vi "prop_axes_main.vi"() -> ()   [LabVIEW 2020, in "3DPC_SurfacePlot.xctl"]
uses:
  <vilib>/Native 3D Graph/xcontrol/3DPC_SurfacePlot.xctl
  <vilib>/Native 3D Graph/typedefs/prop_axes_all.ctl
  <vilib>/Native 3D Graph/typedefs/prop_axes_grid.ctl
  <vilib>/Native 3D Graph/typedefs/prop_axes_ticks.ctl
  <vilib>/Native 3D Graph/typedefs/range_cluster.ctl
  <vilib>/Native 3D Graph/typedefs/min_max.ctl
  <vilib>/Native 3D Graph/typedefs/prop_axes_captions.ctl
  <vilib>/Native 3D Graph/typedefs/prop_axes_labels.ctl
  <vilib>/Native 3D Graph/typedefs/prop_axes_autorange.ctl
  <vilib>/Utility/miscctls.llb/LVPointTypeDef.ctl
panel:
  in  "done":refnum<user-event>
  in  "quit":refnum<user-event>
  out "Axes Properties Out":T1
  in  "Axes Properties In":T1
  in  "Axes Listbox":i32(listbox) caption="Axes"
  in  "Tab Grid Prop":T9(tab)
  in  "Caption Opposite Visibility":bool
  in  "Caption Visibility":bool
  in  "Caption Font Size":i32 caption="Font Size"
  in  "Caption Color":u32(colorbox) caption="Color"
  in  "Caption Text":string
  in  "Label Opposite Visibility":bool
  in  "Label Color":u32(colorbox) caption="Color"
  in  "Label Font Size":i32 caption="Font Size"
  in  "Label Visibility":bool
  in  "Range Auto":bool
  in  "Range Minimum":dbl caption="Minimum"
  in  "Range Maximum":dbl caption="Maximum"
  in  "Grid Visibility":bool
  in  "Grid Color":u32(colorbox) caption="Color"
  in  "Major Tick Visibility":bool
  in  "Tick Color":u32(colorbox) caption="Color"
  in  "Major Tick Count":i32 caption="Count"
  in  "Minor Tick Visibility":bool
  in  "Minor Tick Count":i32 caption="Count"
  out "Boolean":bool caption="Major Ticks"
  out "Boolean 2":bool caption="Minor Ticks"
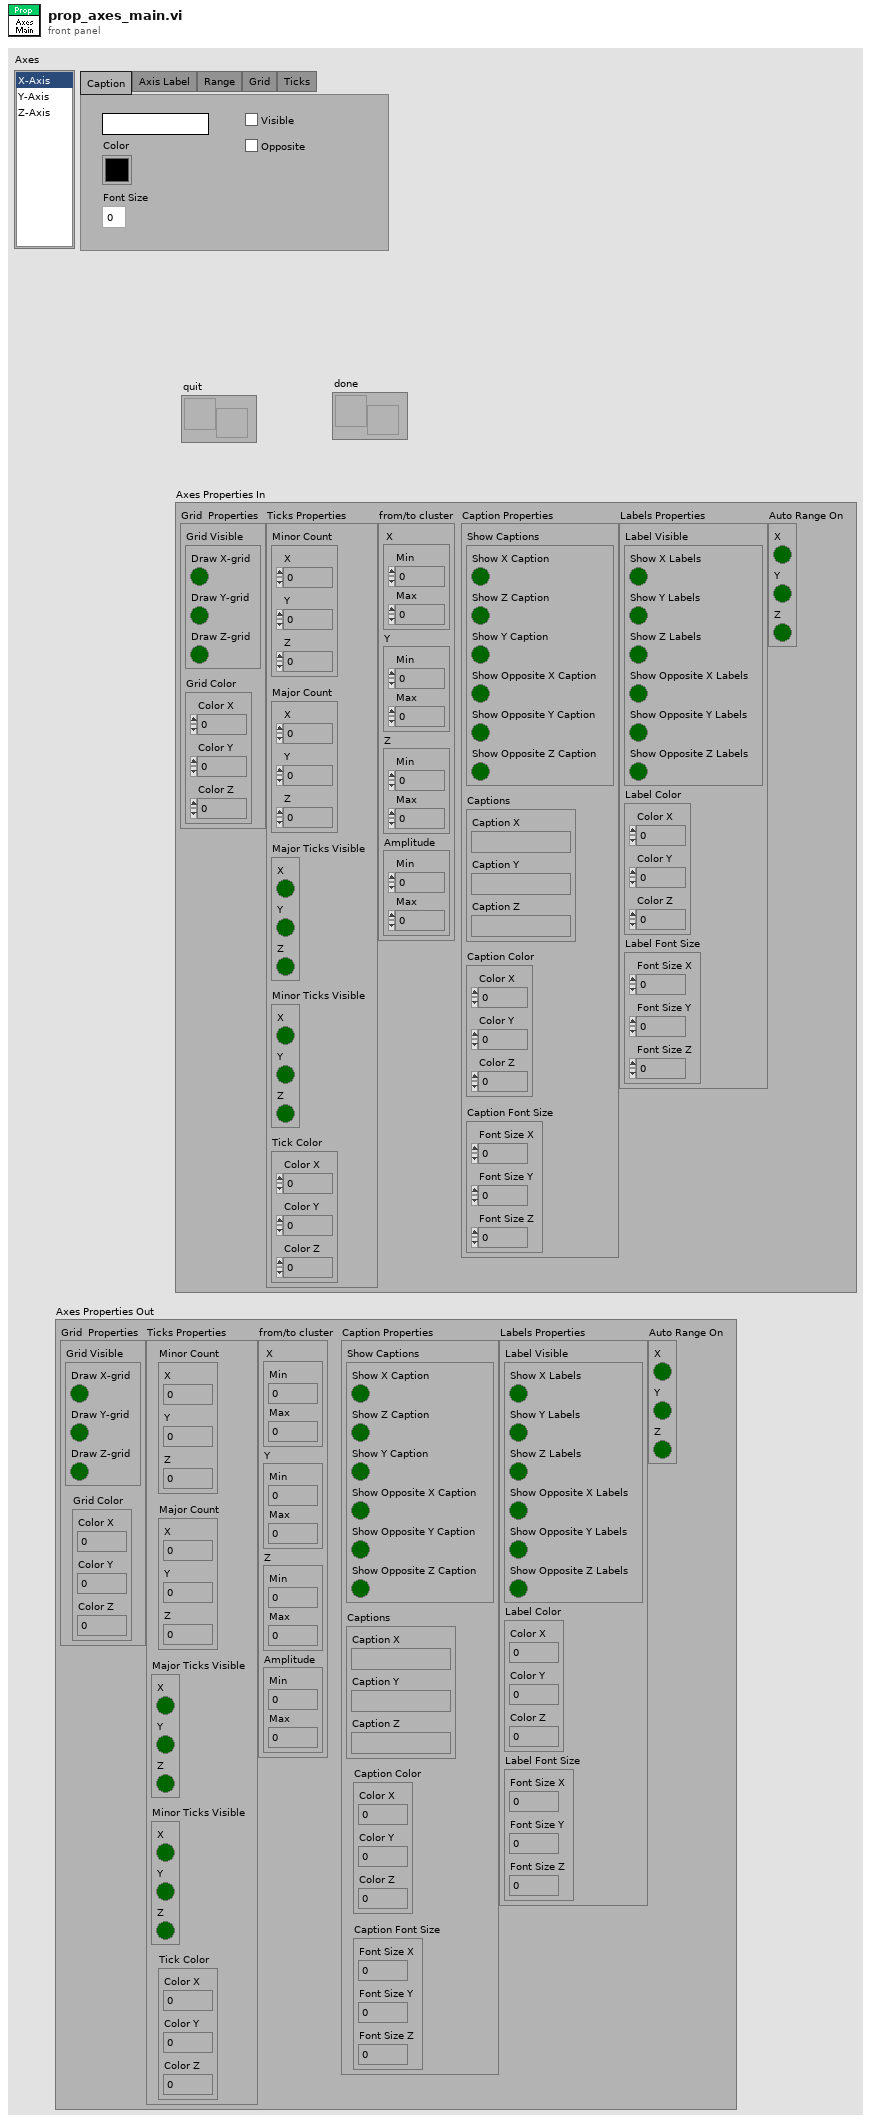
[diagram p1: front panel]
types:
  T1 = typedef "3DPC_SurfacePlot.xctl/prop_axes_all.ctl" = cluster{"Grid  Properties":T2, "Ticks Properties":T3, "from/to cluster":T4, "Caption Properties":T6, "Labels Properties":T7, "Auto Range On":T8}
  T2 = typedef "3DPC_SurfacePlot.xctl/prop_axes_grid.ctl" = cluster{"Grid Visible":cluster{"Draw X-grid":bool, "Draw Y-grid":bool, "Draw Z-grid":bool}, "Grid Color":cluster{"Color X":u32, "Color Y":u32, "Color Z":u32}}
  T3 = typedef "3DPC_SurfacePlot.xctl/prop_axes_ticks.ctl" = cluster{"Minor Count":cluster{"X":i32, "Y":i32, "Z":i32}, "Major Count":cluster{"X":i32, "Y":i32, "Z":i32}, "Major Ticks Visible":cluster{"X":bool, "Y":bool, "Z":bool}, "Minor Ticks Visible":cluster{"X":bool, "Y":bool, "Z":bool}, "Tick Color":cluster{"Color X":u32, "Color Y":u32, "Color Z":u32}}
  T4 = typedef "3DPC_SurfacePlot.xctl/range_cluster.ctl" = cluster{"X":T5, "Y":T5, "Z":T5, "Amplitude":T5}
  T5 = typedef "3DPC_SurfacePlot.xctl/min_max.ctl" = cluster{"Min":sgl, "Max":sgl}
  T6 = typedef "3DPC_SurfacePlot.xctl/prop_axes_captions.ctl" = cluster{"Show Captions":cluster{"Show X Caption":bool, "Show Z Caption":bool, "Show Y Caption":bool, "Show Opposite X Caption":bool, "Show Opposite Y Caption":bool, "Show Opposite Z Caption":bool}, "Captions":cluster{"Caption X":string, "Caption Y":string, "Caption Z":string}, "Caption Color":cluster{"Color X":u32, "Color Y":u32, "Color Z":u32}, "Caption Font Size":cluster{"Font Size X":i16, "Font Size Y":i16, "Font Size Z":i16}}
  T7 = typedef "3DPC_SurfacePlot.xctl/prop_axes_labels.ctl" = cluster{"Label Visible":cluster{"Show X Labels":bool, "Show Y Labels":bool, "Show Z Labels":bool, "Show Opposite X Labels":bool, "Show Opposite Y Labels":bool, "Show Opposite Z Labels":bool}, "Label Color":cluster{"Color X":u32, "Color Y":u32, "Color Z":u32}, "Label Font Size":cluster{"Font Size X":i16, "Font Size Y":i16, "Font Size Z":i16}}
  T8 = typedef "3DPC_SurfacePlot.xctl/prop_axes_autorange.ctl" = cluster{"X":bool, "Y":bool, "Z":bool}
  T9 = enum32{"Caption", "Axis Label", "Range", "Grid", "Ticks"}
  T10 = typedef "LVPointTypeDef.ctl" = cluster{"Horizontal":i16, "Vertical":i16}
  T11 = cluster{"Caption Properties":cluster{"Caption Visibility":bool, "Caption Opposite Visibility":bool, "Caption Color":u32, "Caption Font Size":i32, "Caption Text":string}, "Range Properties":cluster{"Range Auto":bool, "Range Maximum":dbl, "Range Minimum":dbl}, "Grid Properties":cluster{"Grid Visibility":bool, "Grid Color":u32}, "Minor Tick Properties":cluster{"Minor Tick Visibility":bool, "Minor Tick Count":i32}, "Major Tick Properties":cluster{"Major Tick Visibility":bool, "Major Tick Count":i32}, "Label Properties":cluster{"Label Visibility":bool, "Label Opposite Visibility":bool, "Label Color":u32, "Label Font Size":i32}, "Tick Color":u32}[]
  T12 = cluster{"Caption Properties":cluster{"Caption Visibility":bool, "Caption Opposite Visibility":bool, "Caption Color":u32, "Caption Font Size":i32, "Caption Text":string}, "Range Properties":cluster{"Range Auto":bool, "Range Maximum":dbl, "Range Minimum":dbl}, "Grid Properties":cluster{"Grid Visibility":bool, "Grid Color":u32}, "Minor Tick Properties":cluster{"Minor Tick Visibility":bool, "Minor Tick Count":i32}, "Major Tick Properties":cluster{"Major Tick Visibility":bool, "Major Tick Count":i32}, "Label Properties":cluster{"Label Visibility":bool, "Label Opposite Visibility":bool, "Label Color":u32, "Label Font Size":i32}, "Tick Color":u32}
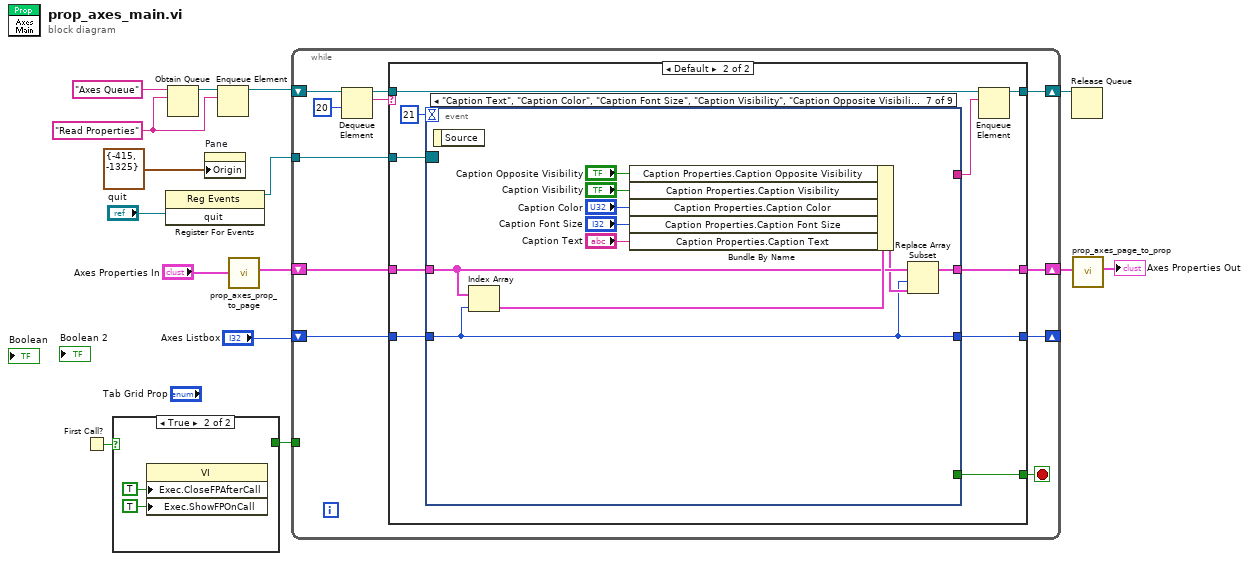
[diagram p0: block diagram]
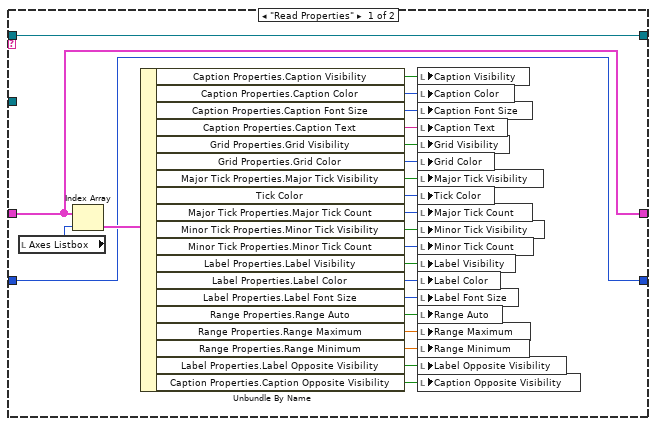
[diagram p2: hidden frame]
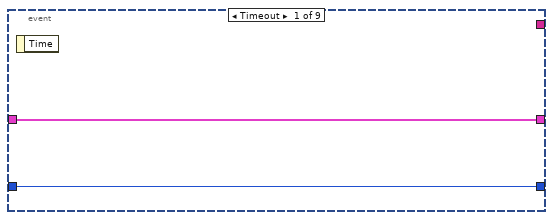
[diagram p3: hidden frame]
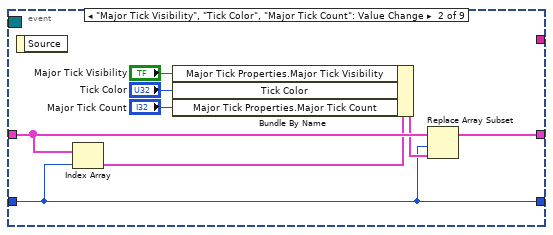
[diagram p4: hidden frame]
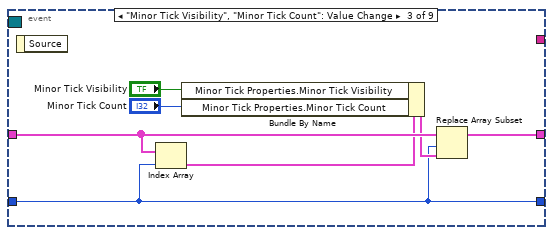
[diagram p5: hidden frame]
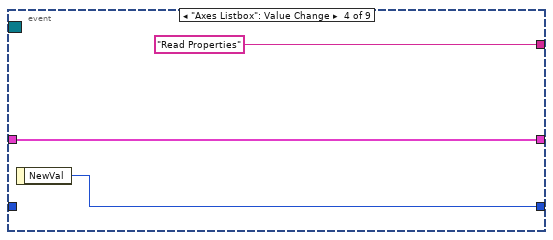
[diagram p6: hidden frame]
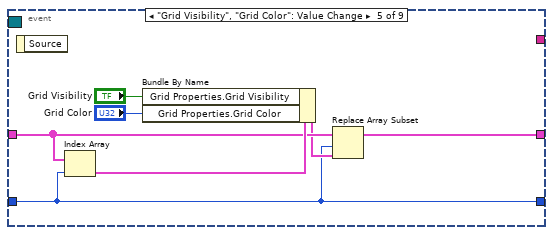
[diagram p7: hidden frame]
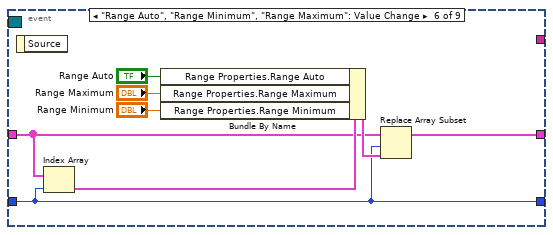
[diagram p8: hidden frame]
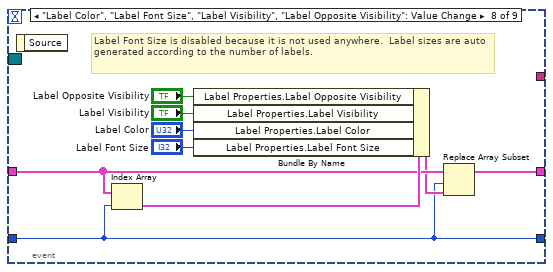
[diagram p9: hidden frame]
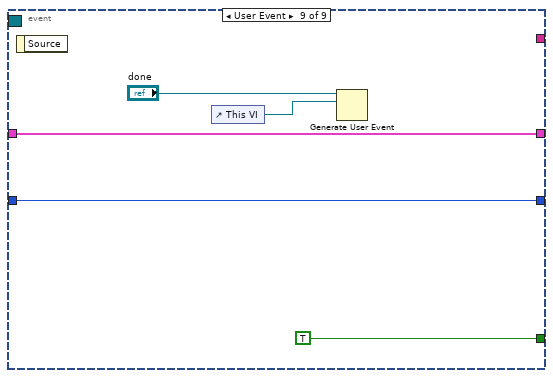
[diagram p10: hidden frame]
diagram:
  w13 = "Read Properties"
  n1 = First Call?() -> (First Call?: T/F=w1:bool)
  n2 = case shown="True" w1 {
    selector: w1 -> [w16 _]
    tunnel: [w16 _] -> w10
    frame False {
    }
    frame True {
      n3 = property class="VI"("Exec.CloseFPAfterCall"=TRUE ("Execution:Close After Call"), "Exec.ShowFPOnCall"=TRUE ("Execution:Show Front Panel On Call")) -> ()  [unwired: 2 in, 2 out]
    }
  }
  n4 = register-events("quit") -> (reference out=w4:refnum<event-registration>)  [unwired: 2 in, 1 out]
  n5 = Obtain Queue(name (unnamed)="Axes Queue", element data type=w13) -> (queue out=w14:refnum<queue>)  [unwired: 3 in, 2 out]
  n6 = property on="Pane" class="Pane"("Origin"=T10 {"Horizontal"=-415, "Vertical"=-1325} ("Point")) -> ()  [unwired: 2 in, 2 out]
  n7 = Enqueue Element(queue=w14, element=w13) -> (queue out=w12:refnum<queue>)  [unwired: 1 in, 3 out]
  n8 = call <vilib>:"prop_axes_prop_to_page.vi"("Axes Properties"="Axes Properties In") -> ("Axes Property Page"=w9:T11)  [unwired: 10 out]
  n9 = while {
    shift-right: [w28] -> w6
    shift-left: w9 -> [w29]
    shift-right: [w24] -> w11
    shift-left: w12 -> [w26]
    tunnel: w10 -> [_]
    tunnel: w4 -> [w22]
    shift-right: [w20] -> _
    shift-left: "Axes Listbox" -> [w19]
    stop <- w21 stop-if-true
    n10 = Dequeue Element(queue=w26, timeout in ms (-1)=20) -> (queue out=w25:refnum<queue>, element=w23:string)  [unwired: 1 in, 2 out]
    n11 = case shown="Default" w23 {
      tunnel: w29 -> [w31 w63]
      tunnel: [w31 w62] -> w28
      tunnel: w25 -> [w53 w60]
      tunnel: [w53 w61] -> w24
      tunnel: w22 -> [_ w57]
      tunnel: [_ w56] -> w21
      tunnel: [w30 w55] -> w20
      tunnel: w19 -> [w30 w54]
      frame "Read Properties" {
        n12 = local read "Axes Listbox"() -> (w32:i32)
        n13 = Index Array(array=w31, index=w32) -> (element=w52:T12)
        n14 = Unbundle By Name(w52) -> ("Caption Properties.Caption Visibility"=w51:bool, "Caption Properties.Caption Color"=w50:u32, "Caption Properties.Caption Font Size"=w49:i32, "Caption Properties.Caption Text"=w48:string, "Grid Properties.Grid Visibility"=w47:bool, "Grid Properties.Grid Color"=w46:u32, "Major Tick Properties.Major Tick Visibility"=w45:bool, "Tick Color"=w44:u32, "Major Tick Properties.Major Tick Count"=w43:i32, "Minor Tick Properties.Minor Tick Visibility"=w42:bool, "Minor Tick Properties.Minor Tick Count"=w41:i32, "Label Properties.Label Visibility"=w40:bool, "Label Properties.Label Color"=w39:u32, "Label Properties.Label Font Size"=w38:i32, "Range Properties.Range Auto"=w37:bool, "Range Properties.Range Maximum"=w36:dbl, "Range Properties.Range Minimum"=w35:dbl, "Label Properties.Label Opposite Visibility"=w34:bool, "Caption Properties.Caption Opposite Visibility"=w33:bool)
        n15 = local write "Caption Visibility"(w51) -> ()
        n16 = local write "Caption Color"(w50) -> ()
        n17 = local write "Caption Font Size"(w49) -> ()
        n18 = local write "Caption Text"(w48) -> ()
        n19 = local write "Grid Visibility"(w47) -> ()
        n20 = local write "Grid Color"(w46) -> ()
        n21 = local write "Major Tick Visibility"(w45) -> ()
        n22 = local write "Tick Color"(w44) -> ()
        n23 = local write "Major Tick Count"(w43) -> ()
        n24 = local write "Minor Tick Visibility"(w42) -> ()
        n25 = local write "Minor Tick Count"(w41) -> ()
        n26 = local write "Label Visibility"(w40) -> ()
        n27 = local write "Label Color"(w39) -> ()
        n28 = local write "Label Font Size"(w38) -> ()
        n29 = local write "Range Auto"(w37) -> ()
        n30 = local write "Range Maximum"(w36) -> ()
        n31 = local write "Range Minimum"(w35) -> ()
        n32 = local write "Label Opposite Visibility"(w34) -> ()
        n33 = local write "Caption Opposite Visibility"(w33) -> ()
      }
      frame Default {
        n34 = event shown="[6] \"Caption Text\", \"Caption Color\", \"Caption Font Size\", \"Caption Visibility\", \"Caption Opposite Visibility\": Value Change" {
          selector: w57 -> [_ _ _ _ _ _ _ _ _]
          dyn-events: _ -> [_ _ _ _ _ _ _ _ _]
          timeout: 21 -> [_ _ _ _ _ _ _ _ _]
          tunnel: w63 -> [w65 w72 w80 w82 w89 w91 w103 w113 w119]
          tunnel: [w65 w73 w75 w82 w88 w97 w101 w111 w119] -> w62
          tunnel: [_ _ _ "Read Properties" _ _ _ _ _] -> w59
          tunnel: [_ _ _ _ _ _ _ _ TRUE] -> w56
          tunnel: [w64 w67 w74 w81 w84 w92 w99 w109 w118] -> w55
          tunnel: w54 -> [w64 w67 w74 _ w84 w92 w99 w109 w118]
          event Timeout {
            n35 = event-data() -> ()  [unwired: 2 out]
          }
          event "Major Tick Visibility", "Tick Color", "Major Tick Count": Value Change {
            n36 = event-data() -> ()  [unwired: 2 out]
            n37 = Index Array(array=w72, index=w67) -> (element=w71:T12)
            n38 = Bundle By Name(cluster=w71, "Major Tick Properties.Major Tick Visibility"="Major Tick Visibility", "Tick Color"="Tick Color", "Major Tick Properties.Major Tick Count"="Major Tick Count") -> (w68:T12)
            n39 = Replace Array Subset(array=w72, new element=w68, index=w67) -> (w73:T11)
          }
          event "Minor Tick Visibility", "Minor Tick Count": Value Change {
            n40 = event-data() -> ()  [unwired: 2 out]
            n41 = Index Array(array=w80, index=w74) -> (element=w79:T12)
            n42 = Bundle By Name(cluster=w79, "Minor Tick Properties.Minor Tick Visibility"="Minor Tick Visibility", "Minor Tick Properties.Minor Tick Count"="Minor Tick Count") -> (w76:T12)
            n43 = Replace Array Subset(array=w80, new element=w76, index=w74) -> (w75:T11)
          }
          event "Axes Listbox": Value Change {
            n44 = event-data() -> ("NewVal"=w81:i32)  [unwired: 1 out]
          }
          event "Grid Visibility", "Grid Color": Value Change {
            n45 = event-data() -> ()  [unwired: 2 out]
            n46 = Index Array(array=w89, index=w84) -> (element=w90:T12)
            n47 = Bundle By Name(cluster=w90, "Grid Properties.Grid Visibility"="Grid Visibility", "Grid Properties.Grid Color"="Grid Color") -> (w87:T12)
            n48 = Replace Array Subset(array=w89, new element=w87, index=w84) -> (w88:T11)
          }
          event "Range Auto", "Range Minimum", "Range Maximum": Value Change {
            n49 = event-data() -> ()  [unwired: 2 out]
            n50 = Index Array(array=w91, index=w92) -> (element=w98:T12)
            n51 = Bundle By Name(cluster=w98, "Range Properties.Range Auto"="Range Auto", "Range Properties.Range Maximum"="Range Maximum", "Range Properties.Range Minimum"="Range Minimum") -> (w93:T12)
            n52 = Replace Array Subset(array=w91, new element=w93, index=w92) -> (w97:T11)
          }
          event "Caption Text", "Caption Color", "Caption Font Size", "Caption Visibility", "Caption Opposite Visibility": Value Change {
            n53 = event-data() -> ()  [unwired: 2 out]
            n54 = Index Array(array=w103, index=w99) -> (element=w104:T12)
            n55 = Bundle By Name(cluster=w104, "Caption Properties.Caption Opposite Visibility"="Caption Opposite Visibility", "Caption Properties.Caption Visibility"="Caption Visibility", "Caption Properties.Caption Color"="Caption Color", "Caption Properties.Caption Font Size"="Caption Font Size", "Caption Properties.Caption Text"="Caption Text") -> (w102:T12)
            n56 = Replace Array Subset(array=w103, new element=w102, index=w99) -> (w101:T11)
          }
          event "Label Color", "Label Font Size", "Label Visibility", "Label Opposite Visibility": Value Change {
            # "Label Font Size is disabled because it is not used anywhere.  Label sizes are auto generated according to the number of labels."
            n57 = event-data() -> ()  [unwired: 2 out]
            n58 = Index Array(array=w113, index=w109) -> (element=w117:T12)
            n59 = Bundle By Name(cluster=w117, "Label Properties.Label Opposite Visibility"="Label Opposite Visibility", "Label Properties.Label Visibility"="Label Visibility", "Label Properties.Label Color"="Label Color", "Label Properties.Label Font Size"="Label Font Size") -> (w112:T12)
            n60 = Replace Array Subset(array=w113, new element=w112, index=w109) -> (w111:T11)
          }
          event User Event {
            n61 = event-data() -> ()  [unwired: 2 out]
            n62 = control-ref of="This VI"() -> (w121:refnum<vi>)
            n63 = Generate User Event(user event="done", event data cluster=w121) -> ()  [unwired: 2 in, 2 out]
          }
        }
        n64 = Enqueue Element(queue=w60, element=w59) -> (queue out=w61:refnum<queue>)  [unwired: 1 in, 3 out]
      }
    }
  }
  n65 = Release Queue(queue=w11) -> ()  [unwired: 1 in, 4 out]
  n66 = call <vilib>:"prop_axes_page_to_prop.vi"("Axes Property Page"=w6) -> ("Axes Properties Out"=→"Axes Properties Out":T1)  [unwired: 10 out]
